vi "Autonomous Independent.vi"   [LabVIEW 2019]
doc: "This VI is called when autonomous begins, and will automatically be terminated when autonomous ends. You can carry out timed or sensor driven robot movement independently without needing to return to the caller."
uses:
  <vilib>/Rock Robotics/Network Tables/NT Read Number.vi
  <vilib>/Rock Robotics/Network Tables/NT Read String.vi
  Robot Global Data.vi
panel:
  # "Be sure to right-click and choose Data Operations>>Make Current Value default if you want to save the array values with the VI"
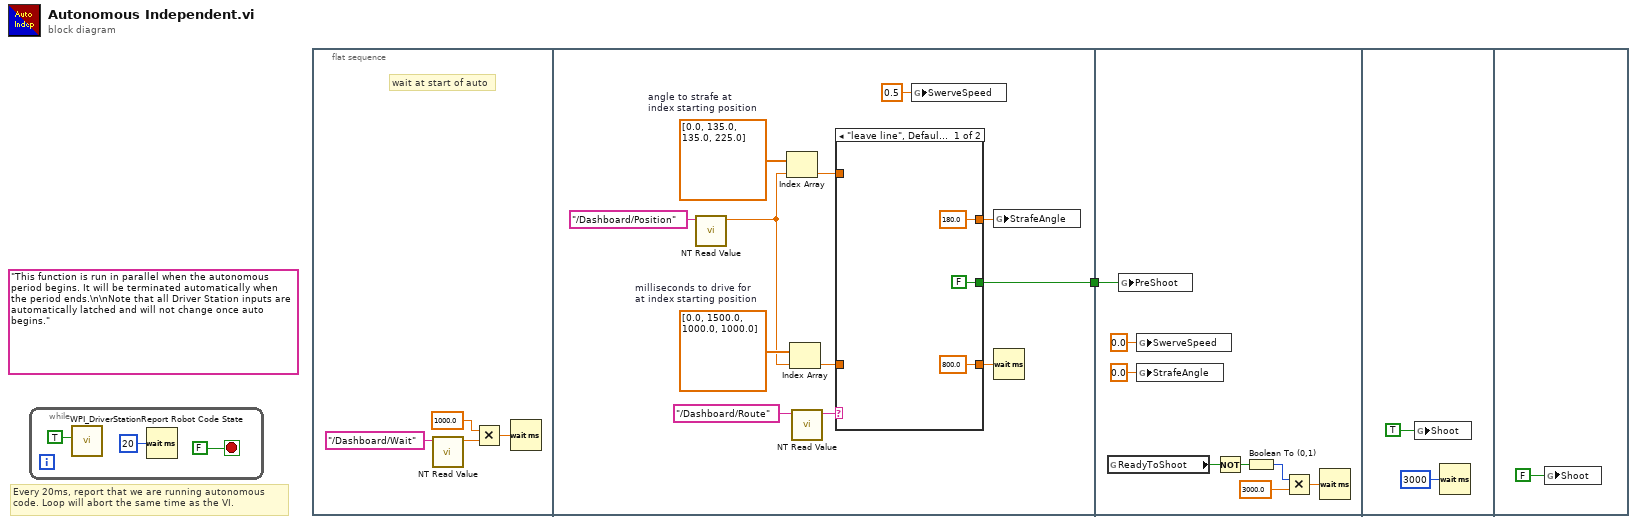
[diagram p0: block diagram]
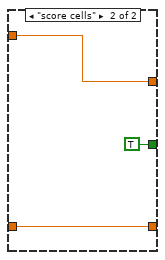
[diagram p2: hidden frame]
diagram:
  (unwired) "This function is run in parallel when the autonomous period begins. It will be terminated automatically when the period ends.\n\nNote that all Driver Station inputs are automatically latched and will not change once auto begins."
  # "Every 20ms, report that we are running autonomous\ncode. Loop will abort the same time as the VI."
  n1 = while {
    stop <- FALSE stop-if-true
    n2 = call <vilib>:"WPI_DriverStationReport Robot Code State.vi"("Autonomous"=TRUE) -> ()  [unwired: 10 in, 1 out]
    n3 = Wait (ms)(milliseconds to wait=u32 20) -> ()  [unwired: 1 out]
  }
  n4 = flat-sequence {
    tunnel: [w9] -> w1
    tunnel: w1 -> [w34]
    frame #0 {
      # "wait at start of auto"
      n5 = call-poly <vilib>:"NT Read Value.vi"("Name"="/Dashboard/Wait") -> ("Numeric"=w7:dbl)  [unwired: 9 in, 1 out]
      n6 = Multiply(x=1000.0, y=w7) -> (x*y=w6:dbl)
      n7 = Wait (ms)(milliseconds to wait=w6) -> ()  [unwired: 1 out]
    }
    frame #1 {
      w12 = dbl[] [0.0, 1500.0, 1000.0, 1000.0]  # milliseconds to drive for at index starting position
      w18 = dbl[] [0.0, 135.0, 135.0, 225.0]  # angle to strafe at index starting position
      n8 = call-poly <vilib>:"NT Read Value.vi"("Name"="/Dashboard/Position") -> ("Numeric"=w11:dbl)  [unwired: 9 in, 1 out]
      n9 = Index Array(array=w18, index=w11) -> (element=w17:dbl)
      n10 = Index Array(array=w12, index=w11) -> (element=w10:dbl)
      n11 = call-poly <vilib>:"NT Read Value.vi"("Name"="/Dashboard/Route") -> ("String"=w16:string)  [unwired: 9 in, 1 out]
      n12 = case shown="\"leave line\", Default" w16 {
        tunnel: [180.0 w26] -> w15
        tunnel: w17 -> [_ w26]
        tunnel: [800.0 w25] -> w13
        tunnel: w10 -> [_ w25]
        tunnel: [FALSE TRUE] -> w9
        frame "leave line", Default {
        }
        frame "score cells" {
        }
      }
      n13 = global write "Robot Global Data.vi" "SwerveSpeed"(0.5 ("SwerveSpeed")) -> ()
      n14 = global write "Robot Global Data.vi" "StrafeAngle"(w15) -> ()
      n15 = Wait (ms)(milliseconds to wait=w13) -> ()  [unwired: 1 out]
    }
    frame #2 {
      n16 = global read "Robot Global Data.vi" "ReadyToShoot"() -> (w31:bool)
      n17 = global write "Robot Global Data.vi" "PreShoot"(w34) -> ()
      n18 = global write "Robot Global Data.vi" "SwerveSpeed"(0.0 ("SwerveSpeed")) -> ()
      n19 = global write "Robot Global Data.vi" "StrafeAngle"(0.0 ("StrafeAngle")) -> ()
      n20 = Not(x=w31) -> (.not. x?=w30:bool)
      n21 = Boolean To (0,1)(Boolean=w30) -> (0, 1=w29:i16)
      n22 = Multiply(x=w29, y=3000.0) -> (x*y=w32:dbl)
      n23 = Wait (ms)(milliseconds to wait=w32) -> ()  [unwired: 1 out]
    }
    frame #3 {
      n24 = global write "Robot Global Data.vi" "Shoot"(TRUE ("Cannon")) -> ()
      n25 = Wait (ms)(milliseconds to wait=u32 3000) -> ()  [unwired: 1 out]
    }
    frame #4 {
      n26 = global write "Robot Global Data.vi" "Shoot"(FALSE ("Cannon")) -> ()
    }
  }
